vi "Handle Messages.vi"(8 "error in (no error)":errorcluster, 9 "Message Data":variant, 10 "Message":string, 11 "Process In":refnum<class "Mock Debug Message Receiver.lvclass">) -> (0 "error out":errorcluster, 3 "Process Out":refnum<class "Mock Debug Message Receiver.lvclass">)   [LabVIEW 2020]
doc: "This is the core VI handling incomming messages to the process. This VI should be overridden to add functionality to the process or override functionality implemented by a parent. Any message not handled should be sent to the parent method using the default case. \nEach state should be atomic and states should in general avoid enqueueing new messages from within this method, as there might be other messages interleaved in the queue from the outside. For cyclic iteration of an action, using a Helper Loop is recommended."
uses:
  Mock Debug Message Receiver.lvclass
  C:/Users/anton/Documents/GitHub/triarc-debugger/source/Process/Debug Process.lvclass
  C:/Users/anton/Documents/GitHub/triarc-debugger/source/Mock Debug Message Receiver.lvclass
  C:/Users/anton/Documents/GitHub/triarc-debugger/source/Debug Data Event/Debug Data Event.lvclass
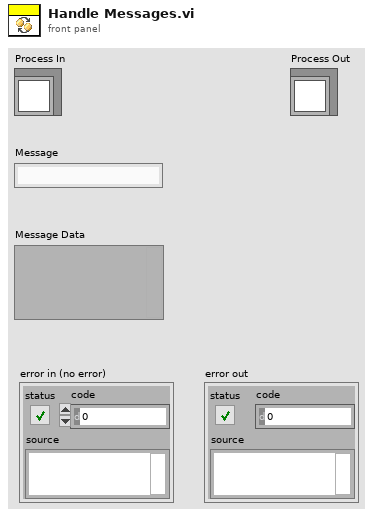
[diagram p1: front panel]
types:
  T1 = cluster{"Action":string, "Call Chain":string, "Process":string, "Message":string, "Message Data":variant, "Time":u32}
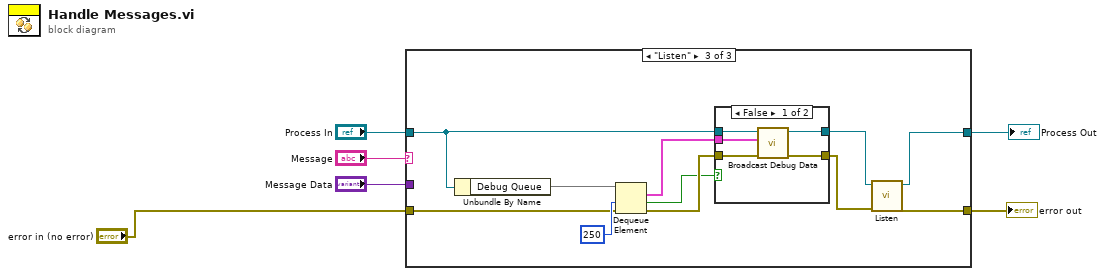
[diagram p0: block diagram]
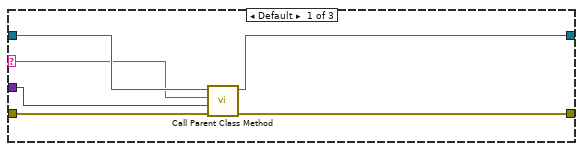
[diagram p2: hidden frame]
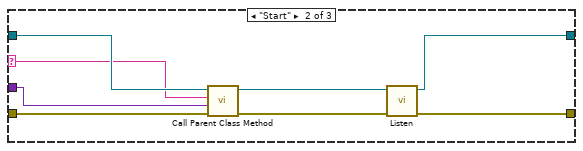
[diagram p3: hidden frame]
diagram:
  n1 = case shown="\"Listen\"" "Message" {
    selector: "Message" -> [w8 w17 _]
    tunnel: "Process In" -> [w10 w18 w27]
    tunnel: [w9 w13 w21] -> w5
    tunnel: [w11 w15 w23] -> w4
    tunnel: "error in (no error)" -> [w12 w20 w25]
    tunnel: "Message Data" -> [w7 w16 _]
    frame Default {
      n2 = call-parent "Call Parent Class Method"("error in (no error)"=w12, "Message Data"=w7, "Message"=w8, "Process In"=w10) -> ("error out"=w11:errorcluster, "Process Out"=w9:refnum<class "Mock Debug Message Receiver.lvclass">)  [unwired: 6 in]
    }
    frame "Start" {
      n3 = call-parent "Call Parent Class Method"("error in (no error)"=w20, "Message Data"=w16, "Message"=w17, "Process In"=w18) -> ("error out"=w19:errorcluster, "Process Out"=w14:refnum<class "Mock Debug Message Receiver.lvclass">)  [unwired: 6 in]
      n4 = call "Listen.vi"("error in (no error)"=w19, "Debug Message Receiver in"=w14) -> ("error out"=w15:errorcluster, "Debug Message Receiver out"=w13:refnum<class "Mock Debug Message Receiver.lvclass">)  [unwired: 8 in]
    }
    frame "Listen" {
      n5 = Unbundle By Name(w27) -> ("Debug Queue"=w26)
      n6 = Dequeue Element(queue=w26, timeout in ms (-1)=250, error in (no error)=w25) -> (element=w30:T1, timed out?=w29:bool, error out=w31:errorcluster)  [unwired: 1 out]
      n7 = case shown="False" w29 {
        tunnel: w30 -> [w33 _]
        tunnel: w27 -> [w36 w37]
        tunnel: w31 -> [w35 w38]
        tunnel: [w34 w38] -> w24
        tunnel: [w32 w37] -> w22
        frame False {
          n8 = call "Broadcast Debug Data.vi"("error in (no error)"=w35, "Debug Data Cluster"=w33, "Debug Message Receiver in"=w36) -> ("error out"=w34:errorcluster, "Debug Message Receiver out"=w32:refnum<class "Mock Debug Message Receiver.lvclass">)  [unwired: 7 in]
        }
        frame True {
        }
      }
      n9 = call "Listen.vi"("error in (no error)"=w24, "Debug Message Receiver in"=w22) -> ("error out"=w23:errorcluster, "Debug Message Receiver out"=w21:refnum<class "Mock Debug Message Receiver.lvclass">)  [unwired: 8 in]
    }
  }
  "error out" <- w4
  "Process Out" <- w5
